vi "Write CurrentFolderShown.vi"(8 "error in (no error)":errorcluster, 10 "CurrentFolderShown":string, 11 "WebBrowser_Mgmt in":refnum<class "WebBrowser_Mgmt.lvclass">) -> (0 "error out":errorcluster, 3 "WebBrowser_Mgmt out":refnum<class "WebBrowser_Mgmt.lvclass">)   [LabVIEW 2016, in "WebBrowser_Mgmt.lvclass"]
uses:
  WebBrowser_Mgmt.lvclass
  WebBrowser_Mgmt.lvclass/WebBrowser_Mgmt.ctl
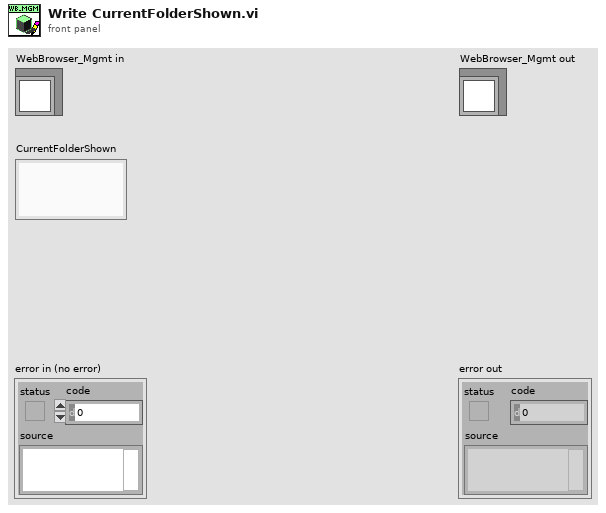
[diagram p1: front panel]
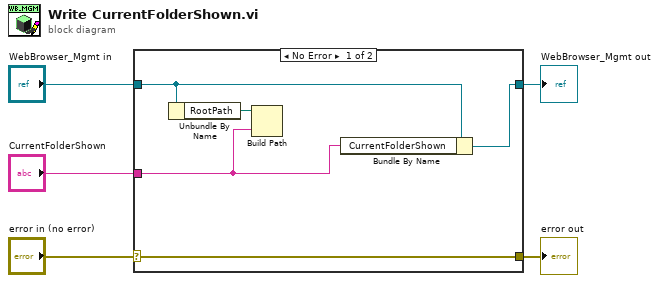
[diagram p0: block diagram]
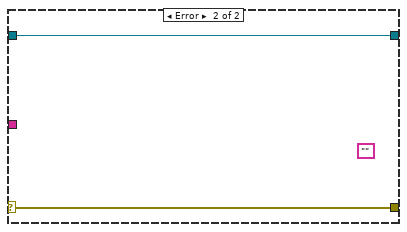
[diagram p2: hidden frame]
diagram:
  n1 = case shown="No Error" "error in (no error)" {
    selector: "error in (no error)" -> [w10 w11]
    tunnel: [w10 w11] -> w4
    tunnel: [w7 w12] -> w2
    tunnel: "WebBrowser_Mgmt in" -> [w9 w12]
    tunnel: "CurrentFolderShown" -> [w6 _]
    frame No Error {
      n2 = Unbundle By Name(w9) -> ("RootPath"=w8:path)
      n3 = Build Path(base path=w8, name or relative path=w6) -> ()  [unwired: 1 out]
      n4 = Bundle By Name(cluster=w9, "CurrentFolderShown"=w6) -> (w7:refnum<class "WebBrowser_Mgmt.lvclass">)
    }
    frame Error {
      (unwired) ""
    }
  }
  "error out" <- w4
  "WebBrowser_Mgmt out" <- w2
